vi "MakeQR Code.vi"(11 "String":string="E4TNS990509T\\25/04/2017\\E4-AC 1965E-170425\\615\\1703-000221") -> (2 "Area Draw":cluster{dbl, dbl}, 3 "QR Code":picture)   [LabVIEW 2016]
uses:
  QR Code Generator v1.1.llb/User Option.ctl
  QR Code Generator v1.1.llb/EC Level.ctl
  <vilib>/picture/picture.llb/Draw 1-Bit Pixmap.vi
  <vilib>/Utility/NIReport.llb/NI_report.lvclass
panel:
  in  "stop":bool
  in  "OK Button":bool
  out "QR Size":i32
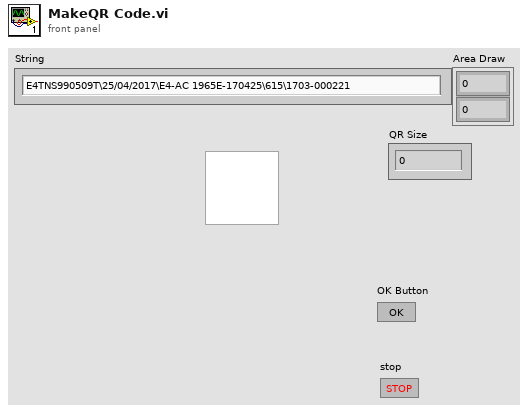
[diagram p1: front panel]
types:
  T1 = typedef "EC Level.ctl" = enum16{"L", "M", "Q", "H"}
  T2 = typedef "User Option.ctl" = enum32{"Automatic", "Numeric", "Alphanumeric", "Plain Text / Website", "Contact Number", "Email Address", "SMS Message"}
  T3 = enum16{"maximized", "minimized", "normal", "no change"}
  T4 = enum16{"Standard Report", "HTML", "Word", "Excel"}
  T5 = cluster{"position (Excel)":cluster{"row":i32, "column":i32}, "name (Excel)":string, "bookmark (Word)":string}
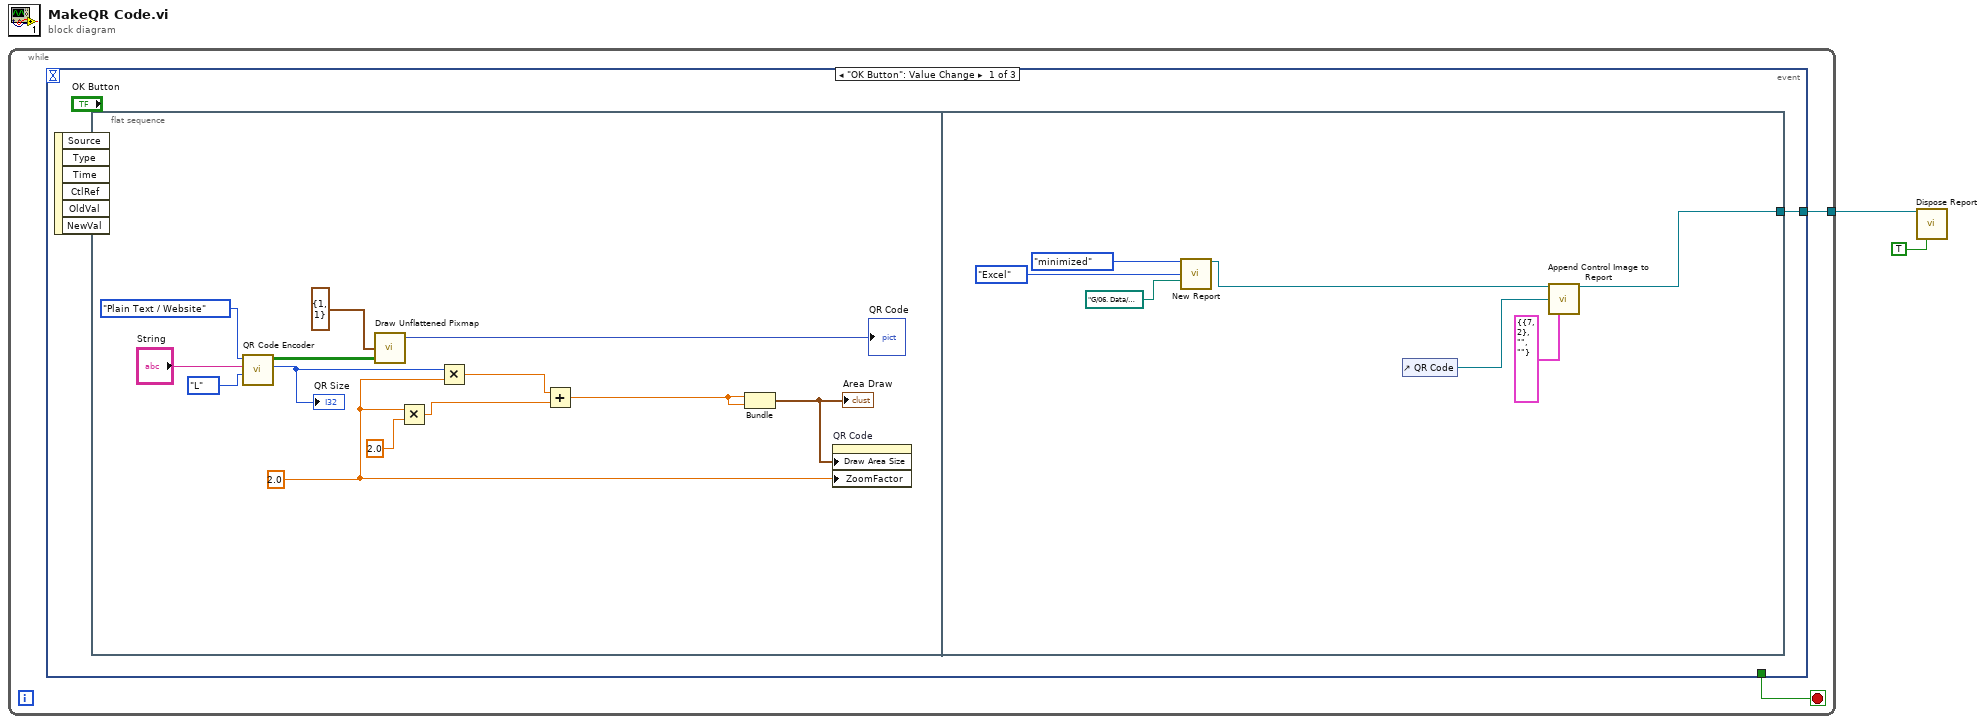
[diagram p0: block diagram]
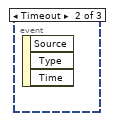
[diagram p2: hidden frame]
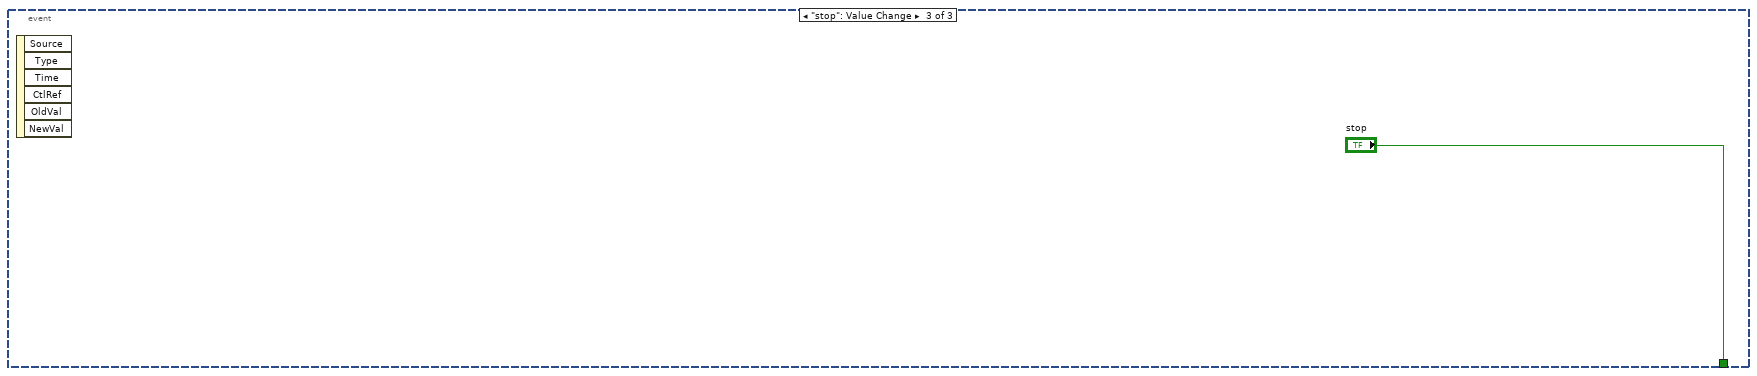
[diagram p3: hidden frame]
diagram:
  n1 = while {
    tunnel: [w4] -> w2
    stop <- w3 stop-if-true
    n2 = event shown="[0] \"OK Button\": Value Change" {
      selector: _ -> [_ _ _]
      dyn-events: _ -> [_ _ _]
      timeout: _ -> [_ _ _]
      tunnel: [w5 _ _] -> w4
      tunnel: [_ _ "stop"] -> w3
      event "OK Button": Value Change {
        n3 = event-data() -> ()  [unwired: 1 in, 6 out]
        n4 = flat-sequence {
          tunnel: [w23] -> w5
          frame #0 {
            w7 = 2.0 ("size")
            n5 = call "QR Code Encoder.vi"("EC Level"=EC_Level."L", "Message"="String", "User Option"=User_Option."Plain Text / Website") -> ("QR Size"=w8:i32, "QR Data"=w16:bool[][])  [unwired: 7 in]
            "QR Size" <- w8
            n6 = call-poly <vilib>:"Draw Unflattened Pixmap.vi"("top left point(0, 0)"=cluster{"x":i16, "y":i16} {"x"=1, "y"=1}, "data"=w16) -> ("new picture"=→"QR Code":picture)  [unwired: 7 in]
            n7 = Multiply(x=w7, y=2.0) -> (x*y=w10:dbl)
            n8 = Multiply(x=w8, y=w7) -> (x*y=w6:dbl)
            n9 = Add(x=w6, y=w10) -> (x+y=w9:dbl)
            n10 = Bundle(w9, w9) -> (w12:cluster{dbl, dbl})  [unwired: 1 in]
            "Area Draw" <- w12
            n11 = property on="QR Code" class="Pict"("Draw Area Size"=w12, "ZoomFactor"=w7) -> ()  [unwired: 2 in, 2 out]
          }
          frame #1 {
            n12 = call <vilib>:"New Report.vi"("window state (normal)"=T3."minimized", "report type"=T4."Excel", "template (empty)"=path "G:/06. Data/Data/05. AEC/07. New Storage Management/Reference/LABEL.xlsx") -> ("report out"=w19:refnum<class "NI_report.lvclass">)  [unwired: 11 in, 1 out]
            n13 = control-ref of="QR Code"() -> (w25:refnum<vi>)
            n14 = call-dynamic "Append Control Image to Report.vi"("report in"=w19, "ctrl reference"=w25, "MS Office parameters"=T5 {"position (Excel)"={"row"=7, "column"=2}, "name (Excel)"="", "bookmark (Word)"=""}) -> ("report out"=w23:refnum<class "NI_report.lvclass">)  [unwired: 9 in, 3 out]
          }
        }
      }
      event Timeout {
        n15 = event-data() -> ()  [unwired: 1 in, 3 out]
      }
      event "stop": Value Change {
        n16 = event-data() -> ()  [unwired: 1 in, 6 out]
      }
    }
  }
  n17 = call-dynamic "Dispose Report.vi"("report in"=w2, "close report? (T)"=TRUE) -> ()  [unwired: 13 in, 1 out]
